vi "ResonanceScanner.vi"() -> ()   [LabVIEW 2012]
uses:
  <vilib>/Platform/TimedLoop/XDataNode/timing_clust.ctl
  <vilib>/Platform/TimedLoop/XDataNode/nitl_modes.ctl
  <vilib>/Platform/TimedLoop/XDataNode/wakeup.ctl
  <vilib>/rvi/eio/common/nirviEmuTemplateMethod_errors.vi
  <vilib>/rvi/FIFO/Fifo_Resource/nirvififoEmulationSetSize.vi
  <vilib>/rvi/DataTransferAndStorage/Container/Common/niFpgaContainerGetUniqueNameForEmu.vi
  <vilib>/rvi/Emulation/niFpgaSctlEmulationRegisterWithScheduler.vi
  <vilib>/rvi/errors/niFpgaSetErrorForExecOnDevCompSimple.vi
  <vilib>/rvi/eio/common/nirviEmuReportErrorAndStop.vi
  <vilib>/rvi/Emulation/niFpgaSctlEmulationFifoFullMgr.vi
  <vilib>/rvi/Emulation/niFpgaSctlEmulationResourceMgr.vi
  <vilib>/rvi/Emulation/niFpgaSctlEmulationScheduler.vi
  <vilib>/rvi/interface/RandomDataEmulation/nirviRandomDataFPGAFIFO.vi
  <vilib>/rvi/interface/RandomDataEmulation/niFpgaRandomDataHandleErrors.vi
  <vilib>/rvi/Emulation/niFpgaSctlEmulationGlobalWrite.vi
  <vilib>/Platform/TimedLoop/XDataNode/XDataNode.xnode
  <vilib>/eio/EIONode/EIONode.xnode
  <vilib>/rvi/DataTransferAndStorage/Container/XNode/niFpgaContainer.xnode
  <vilib>/rvi/FIFO/Fifo_Resource/nirvififoEmulationClear.vi
  <vilib>/rvi/FXPMathLib/basic elements/FxpDiscreteDelay/XNode/nifxpmath_DiscreteDelay.xnode
  <vilib>/rvi/FIFO/Fifo_Resource/nirvififoEmulationWrite.vi
  <vilib>/rvi/FIFO/Fifo_Resource/nirvififoEmulationRead.vi
  <vilib>/rvi/interface/RandomDataEmulation/nirviRandomDataFpgaReadWriteTemplate.vi
  <vilib>/Platform/TimedLoop/XDataNode/XDNodeRunTimeDep.lvlib
panel:
  in  "Scanner delay":i16=10000
  out "Pixel finished?":bool
  out "Resonance Trigger":bool
  in  "Baselinex8 Ch2":u16
  in  "Baselinex8 Ch1":u16
  in  "Clear Interloop FIFO":bool
  out "InterloopFIFO Timeout":bool
  out "ToHostCh2FIFO Overflow":bool
  out "ToHostCh1FIFO Overflow":bool
  out "Pixel counter":u32
  in  "Wait for trigger":bool
  in  "Acquire":bool
  in  "Acquire continuously":bool=TRUE
  in  "Requested pixels":u32=100000
  out "InterloopFIFO Overflow":bool
  out "Acquiring":bool
  out "IO Module\\AI Over Range":bool
  in  "Samples per pixel":u32=10000 caption="Samples per pixel Acq"
  in  "Samples per line":u32=10000 caption="Samples per pixel Acq"
  out "Configured?":bool
  # "5751 IO module configuration"
  # "Analog integrator"
  # "Acquisition control"
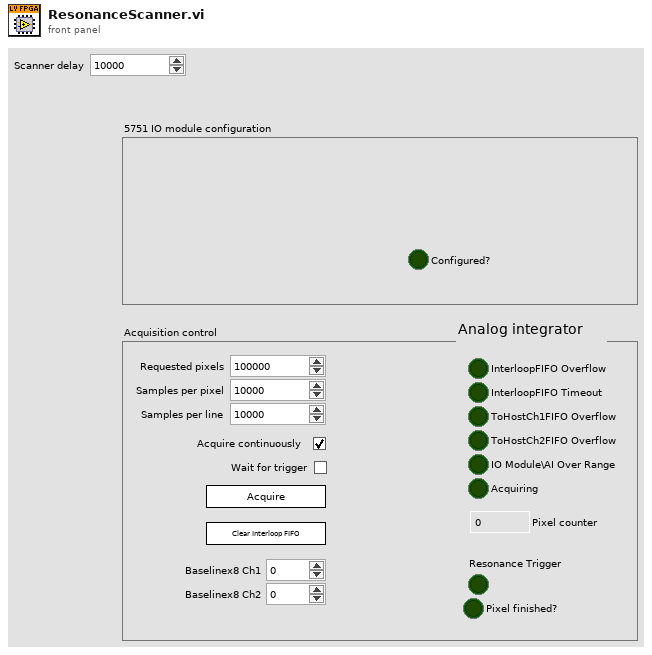
[diagram p1: front panel]
types:
  T1 = typedef "XDNodeRunTimeDep.lvlib/timing_clust.ctl" = cluster{"Expected End [f-1]":u64, "Actual End [f-1]":u64, "Finished Late? [f-1]":bool, "Expected End [i-1]":u64, "Actual End [i-1]":u64, "Finished Late? [i-1]":bool, "Expected Start [i]":u64, "Actual Start [i]":u64, "Expected Start [f]":u64, "Actual Start [f]":u64, "Source Name":string, "Structure Name":string, "Period":i64, "Deadline":i64, "Offset":i64, "Start":i64, "Priority":i32, "Timeout":i32, "Mode":T2, "Wakeup Reason":T3, "Error":errorcluster, "Source Type":string, "Secondary Source Type":string, "Global End Time":u64, "Global Start Time":u64, "Frame Duration":u64, "Iteration Duration":u64, "Assigned CPU":i32, "I/O Scan Engine Mode":u32}
  T2 = typedef "XDNodeRunTimeDep.lvlib/nitl_modes.ctl" = enum32{"No Change", "Process missed periods, maintain original phase", "Discard missed periods, maintain original phase", "Process missed periods, ignore original phase", "Discard missed periods, ignore original phase"}
  T3 = typedef "XDNodeRunTimeDep.lvlib/wakeup.ctl" = enum32{"Normal", "Aborted", "Asynchronous wakeup", "Timing source error", "Timed loop error", "Timeout"}
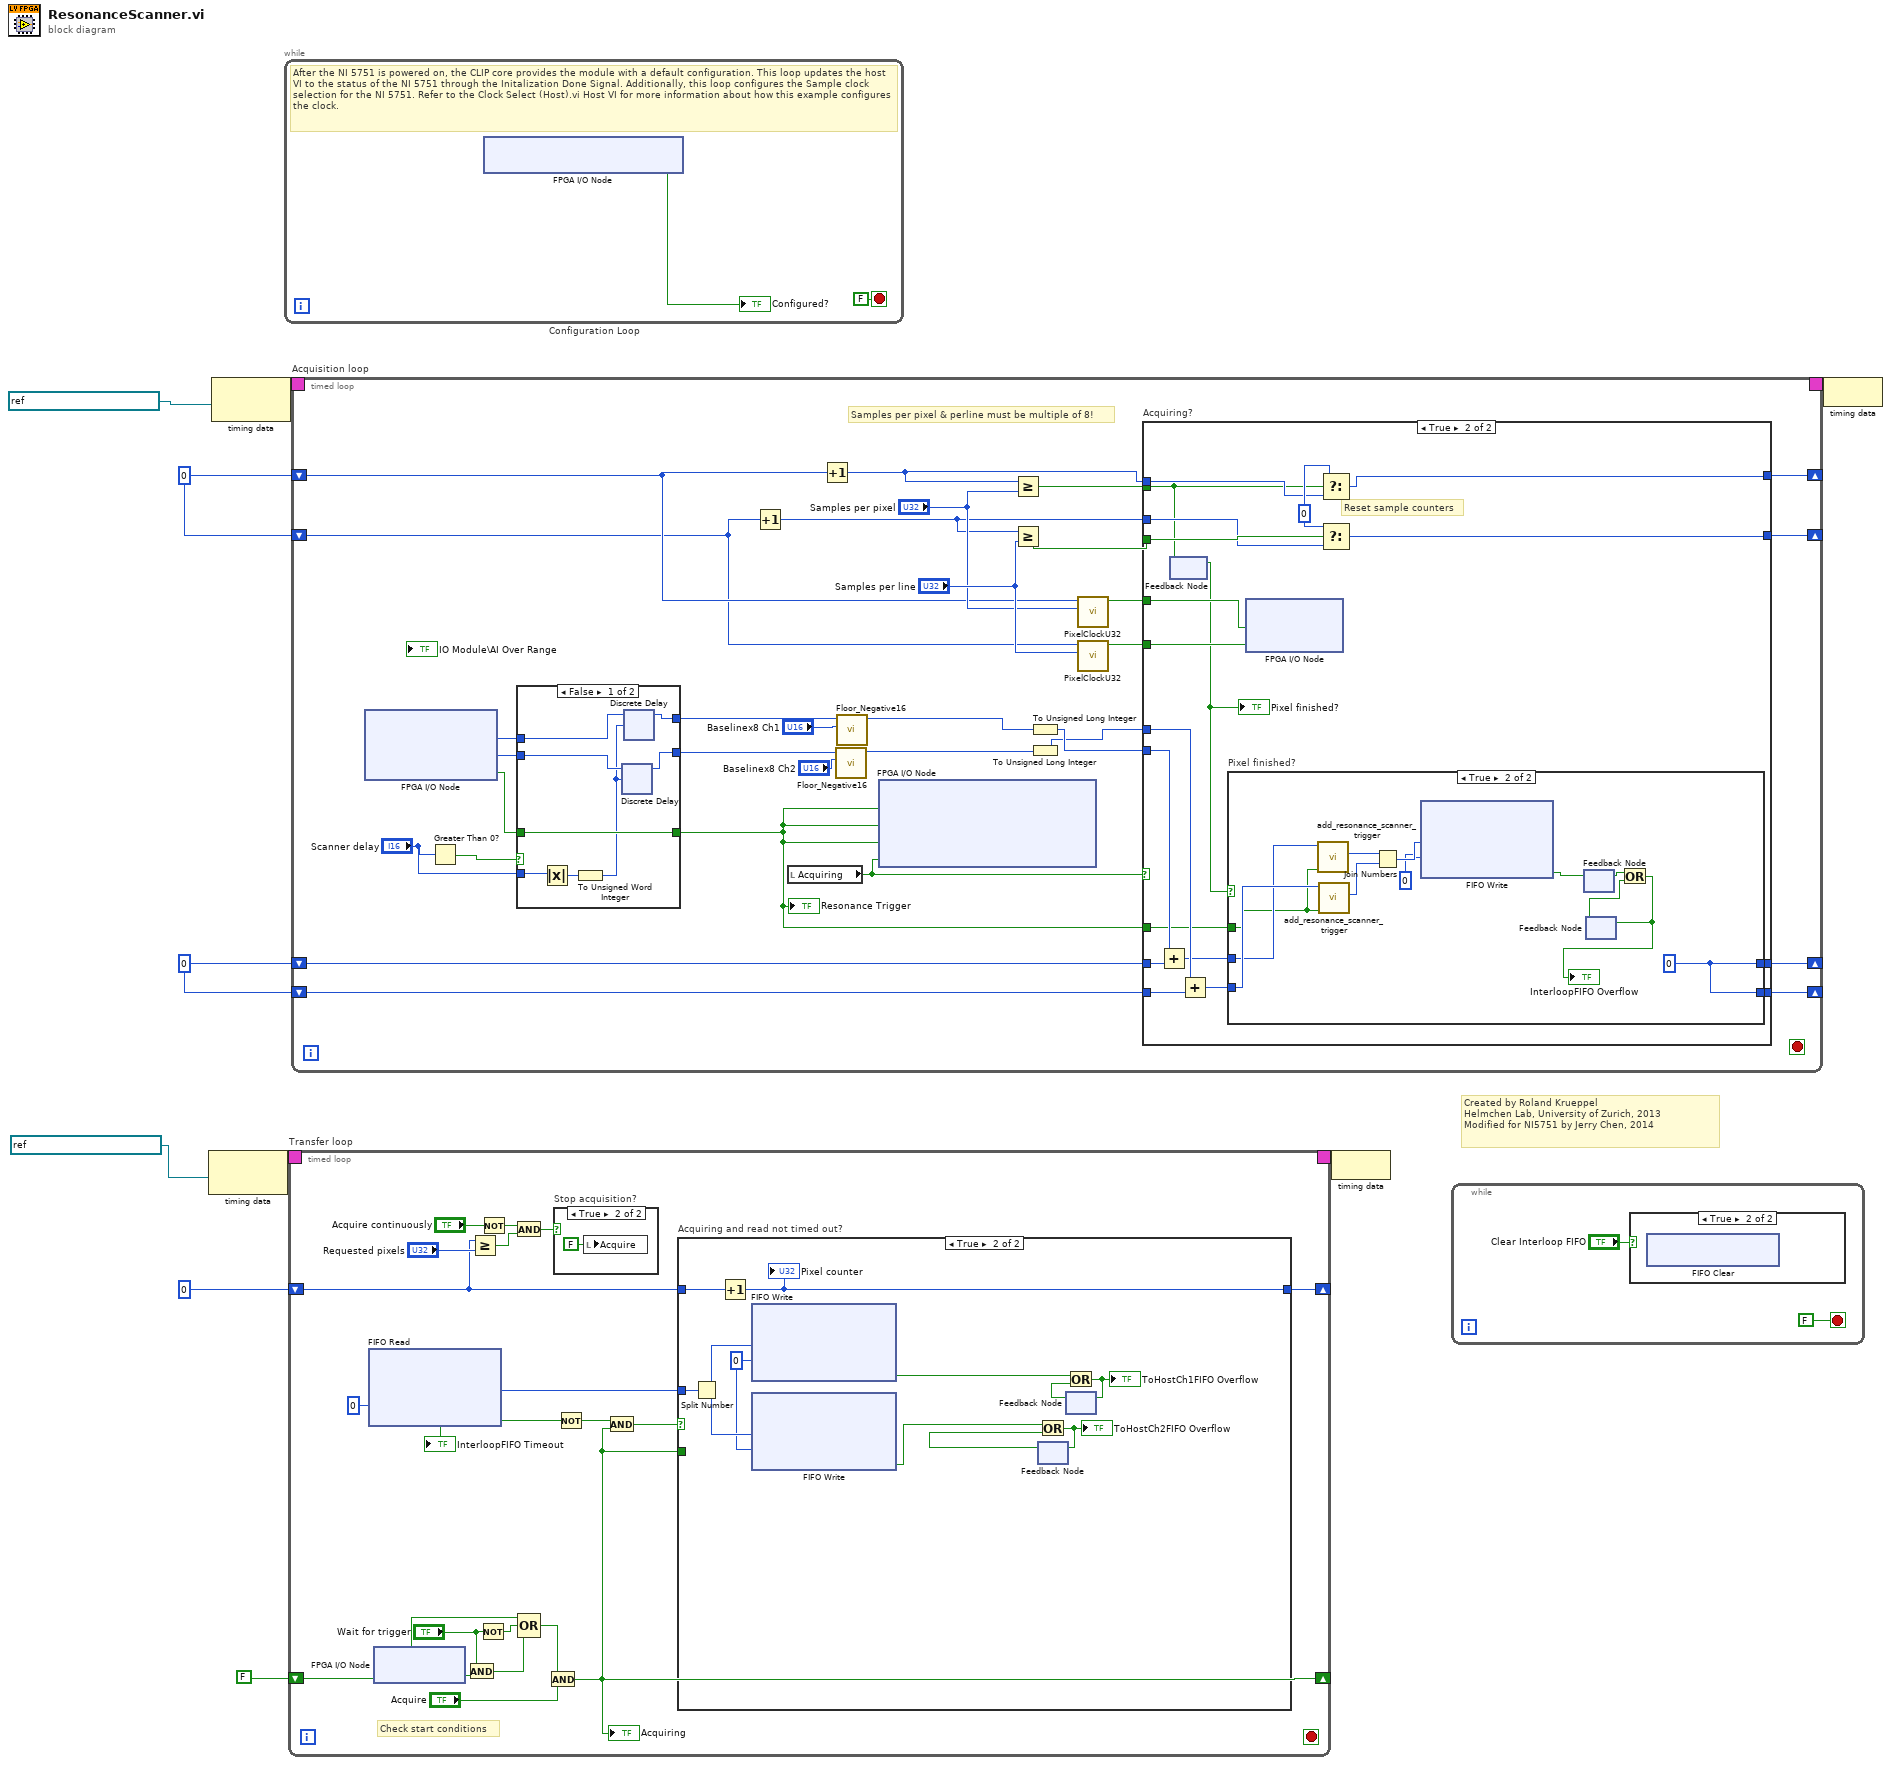
[diagram p0: block diagram]
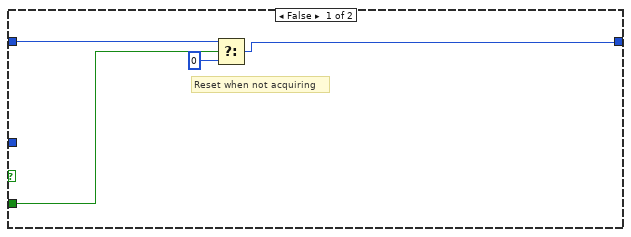
[diagram p4: hidden frame]
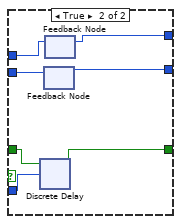
[diagram p5: hidden frame]
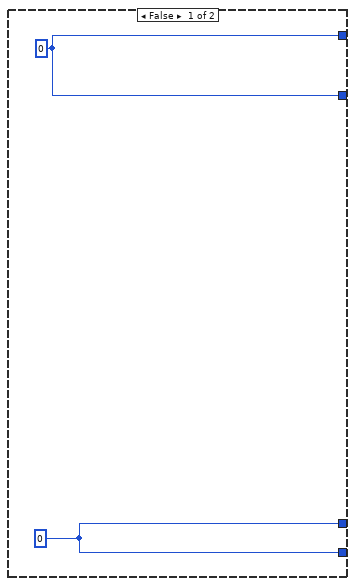
[diagram p6: hidden frame]
diagram:
  w7 = u32 0
  w8 = u32 0 ("t")
  # "Created by Roland Krueppel\nHelmchen Lab, University of Zurich, 2013\nModified for NI5751 by Jerry Chen, 2014"
  n1 = node-c288(refnum<k21> "40 MHz Onboard Clock" ("Source Name")) -> (w6:T1)
  n2 = node-c288(refnum<k21> "40 MHz Onboard Clock" ("Source Name")) -> (w10:T1)
  n3 = while "Configuration Loop" {
    stop <- FALSE stop-if-true
    # "After the NI 5751 is powered on, the CLIP core provides the module with a default configuration. This loop updates the host VI to the status of the NI 5751 through the Initalization Done Signal. Additionally, this loop configures the Sample clock selection for the NI 5751. Refer to the Clock Select (Host).vi Host VI for more information about how this example configures the clock."
    n4 = xnode "FPGA I/O Node"() -> ("IO Module\\Initialization Done"=→"Configured?":bool)  [unwired: 1 in, 1 out]
  }
  n5 = timed-loop "Transfer loop" {
    timing: w6 -> [_]
    timing-out: [_] -> w5
    shift-right: [w15] -> _
    shift-left: u32 0 -> [w16]
    shift-right: [w14] -> _
    shift-left: FALSE -> [w22]
    stop <- _ stop-if-true
    # "Check start conditions"
    n6 = xnode ("FIFO Read")("Timeout"=0) -> ("Element"=w17:u64, "Timed Out?"=w21:bool)  [unwired: 1 in, 1 out]
    "InterloopFIFO Timeout" <- w21
    n7 = xnode "FPGA I/O Node"() -> ("TriggerIn"=w27:bool)  [unwired: 1 in, 1 out]
    n8 = And(x="Wait for trigger", y=w27) -> (x .and. y?=w24:bool)
    n9 = Greater Or Equal?(x=w16, y="Requested pixels") -> (x >= y?=w29:bool)
    n10 = Not(x="Wait for trigger") -> (.not. x?=w25:bool)
    n11 = Not(x="Acquire continuously") -> (.not. x?=w30:bool)
    n12 = And(x=w30, y=w29) -> (x .and. y?=w19:bool)
    n13 = Compound Arithmetic op=OR(w22, w25, w24) -> (w23:bool)
    n14 = And(x=w23, y="Acquire") -> (x .and. y?=w14:bool)
    "Acquiring" <- w14
    n15 = case "Stop acquisition?" shown="True" w19 {
      frame False {
      }
      frame True {
        n16 = local write "Acquire"(FALSE ("Acquire")) -> ()
      }
    }
    n17 = Not(x=w21) -> (.not. x?=w20:bool)
    n18 = And(x=w20, y=w14) -> (x .and. y?=w18:bool)
    n19 = case "Acquiring and read not timed out?" shown="True" w18 {
      tunnel: w17 -> [_ w49]
      tunnel: w16 -> [w36 w45]
      tunnel: [w35 w44] -> w15
      tunnel: w14 -> [w37 _]
      frame False {
        # "Reset when not acquiring"
        n20 = Select(t=w36, s=w37, f=u32 0) -> (s? t:f=w35:u32)
      }
      frame True {
        w46 = 0 ("Timeout")
        n21 = Split Number(x=w49) -> (hi(x)=w48:u32, lo(x)=w47:u32)
        n22 = Increment(x=w45) -> (x+1=w44:u32)
        "Pixel counter" <- w44
        n23 = xnode ("FIFO Write")("Element"=w48, "Timeout"=w46) -> ("Timed Out?"=w42:bool)  [unwired: 1 in, 1 out]
        n24 = xnode ("FIFO Write")("Element"=w47, "Timeout"=w46) -> ("Timed Out?"=w39:bool)  [unwired: 1 in, 1 out]
        n25 = feedback #1() -> (w38:bool)  [unwired: 1 in]
        n26 = Or(x=w39, y=w38) -> (x .or. y?=w40:bool)
        "ToHostCh2FIFO Overflow" <- w40
        n27 = feedback-in #1(w40) -> ()
        n28 = feedback #2() -> (w41:bool)  [unwired: 1 in]
        n29 = Or(x=w42, y=w41) -> (x .or. y?=w43:bool)
        "ToHostCh1FIFO Overflow" <- w43
        n30 = feedback-in #2(w43) -> ()
      }
    }
  }
  n31 = timed-loop "Acquisition loop" {
    timing: w10 -> [_]
    timing-out: [_] -> w9
    shift-right: [w81] -> _
    shift-left: w8 -> [w62]
    shift-right: [w82] -> _
    shift-left: w8 -> [w64]
    shift-right: [w78] -> _
    shift-left: w7 -> [w80]
    shift-right: [w77] -> _
    shift-left: w7 -> [w79]
    stop <- _ stop-if-true
    # "Samples per pixel & perline must be multiple of 8!"
    n32 = xnode "FPGA I/O Node"() -> ("IO Module\\AI A0"=w56:i16, "IO Module\\AI A2"=w55:i16, "IO Module\\DI 0"=w60:bool)  [unwired: 3 in, 3 out]
    n33 = Greater Than 0?(x="Scanner delay") -> (x > 0?=w52:bool)
    n34 = case shown="False" w52 {
      tunnel: w60 -> [w86 w97]
      tunnel: [w86 w96] -> w58
      tunnel: "Scanner delay" -> [w85 w95]
      tunnel: w56 -> [w89 w94]
      tunnel: w55 -> [w90 w93]
      tunnel: [w87 w92] -> w54
      tunnel: [w88 w91] -> w53
      frame False {
        n35 = Absolute Value(x=w85) -> (abs(x)=w84:i16)
        n36 = To Unsigned Word Integer(number=w84) -> (unsigned 16bit integer=w83:u16)
        n37 = xnode "Discrete Delay"("D"=w90, "n-1[0..511]"=w83) -> ("Q"=w87:i16)
        n38 = xnode "Discrete Delay"("D"=w89, "n-1[0..511]"=w83) -> ("Q"=w88:i16)
      }
      frame True {
        n39 = xnode ("Discrete Delay")("D"=w97, "n-1[0..511]"=w95) -> ("Q"=w96:bool)
        n40 = feedback #3() -> (w92:i16)  [unwired: 1 in]
        n41 = feedback-in #3(w93) -> ()
        n42 = feedback #4() -> (w91:i16)  [unwired: 1 in]
        n43 = feedback-in #4(w94) -> ()
      }
    }
    "Resonance Trigger" <- w58
    n44 = Increment(x=w62) -> (x+1=w61:u32)
    n45 = local read "Acquiring"() -> (w59:bool)
    n46 = Increment(x=w64) -> (x+1=w63:u32)
    n47 = call "Floor_Negative16.vi"("Baseline U16"="Baselinex8 Ch2", "Input Value"=w54) -> ("Output Value"=w69:u16)  [unwired: 9 in]
    n48 = call "Floor_Negative16.vi"("Baseline U16"="Baselinex8 Ch1", "Input Value"=w53) -> ("Output Value"=w70:u16)  [unwired: 9 in]
    n49 = xnode "FPGA I/O Node"("IO Module\\D0 2"=w58, "IO Module\\D0 3"=w58, "IO Module\\D0 4"=w58, "IO Module\\Digital Output Enable"=w59) -> ()  [unwired: 4 in, 4 out]
    n50 = Greater Or Equal?(x=w63, y="Samples per pixel") -> (x >= y?=w72:bool)
    n51 = Greater Or Equal?(x=w61, y="Samples per line") -> (x >= y?=w71:bool)
    n52 = To Unsigned Long Integer(number=w70) -> (unsigned 32bit integer=w66:u32)
    n53 = To Unsigned Long Integer(number=w69) -> (unsigned 32bit integer=w65:u32)
    n54 = call "PixelClockU32.vi"("Samples per pixel"="Samples per pixel", "Sample counter"=w64) -> ("Pixel clock"=w74:bool)  [unwired: 9 in]
    n55 = call "PixelClockU32.vi"("Samples per pixel"="Samples per line", "Sample counter"=w62) -> ("Pixel clock"=w73:bool)  [unwired: 9 in]
    n56 = case "Acquiring?" shown="True" w59 {
      tunnel: [w99 w117] -> w82
      tunnel: [w99 w116] -> w81
      tunnel: w66 -> [_ w114]
      tunnel: w80 -> [_ w115]
      tunnel: w79 -> [_ w113]
      tunnel: w65 -> [_ w112]
      tunnel: [w98 w109] -> w78
      tunnel: [w98 w108] -> w77
      tunnel: w72 -> [_ w102]
      tunnel: w71 -> [_ w107]
      tunnel: w63 -> [_ w106]
      tunnel: w61 -> [_ w105]
      tunnel: w74 -> [_ w104]
      tunnel: w73 -> [_ w103]
      tunnel: w58 -> [_ w101]
      frame False {
        w98 = u32 0
        w99 = u16 0 ("t")
      }
      frame True {
        w118 = u32 0 ("t")
        # "Reset sample counters"
        n57 = Add(x=w114, y=w115) -> (x+y=w110:u32)
        n58 = feedback #5() -> (w100:bool)  [unwired: 1 in]
        "Pixel finished?" <- w100
        n59 = feedback-in #5(w102) -> ()
        n60 = Add(x=w112, y=w113) -> (x+y=w111:u32)
        n61 = case "Pixel finished?" shown="True" w100 {
          tunnel: w111 -> [w119 w125]
          tunnel: w110 -> [w120 w124]
          tunnel: [w120 w128] -> w109
          tunnel: [w119 w128] -> w108
          tunnel: w101 -> [_ w123]
          frame False {
          }
          frame True {
            w128 = u32 0
            n62 = call "add_resonance_scanner_trigger.vi"("Trigger"=w123, "Input"=w124) -> ("Output"=w122:u32)  [unwired: 9 in]
            n63 = call "add_resonance_scanner_trigger.vi"("Trigger"=w123, "Input"=w125) -> ("Output"=w121:u32)  [unwired: 9 in]
            n64 = Join Numbers(hi=w122, lo=w121) -> ((hi.lo)=w132:u64)
            n65 = xnode ("FIFO Write")("Element"=w132, "Timeout"=0) -> ("Timed Out?"=w126:bool)  [unwired: 1 in, 1 out]
            n66 = feedback-in #6(w126) -> ()
            n67 = feedback #6() -> (w127:bool)  [unwired: 1 in]
            n68 = feedback #7() -> (w129:bool)  [unwired: 1 in]
            n69 = Or(x=w127, y=w129) -> (x .or. y?=w130:bool)
            "InterloopFIFO Overflow" <- w130
            n70 = feedback-in #7(w130) -> ()
          }
        }
        n71 = xnode "FPGA I/O Node"("PixelClock"=w104, "LineClock"=w103) -> ()  [unwired: 2 in, 2 out]
        n72 = Select(t=w118, s=w102, f=w106) -> (s? t:f=w117:u32)
        n73 = Select(t=w118, s=w107, f=w105) -> (s? t:f=w116:u32)
      }
    }
  }
  n74 = node-c288(w5) -> ()
  n75 = while {
    stop <- FALSE stop-if-true
    n76 = case shown="True" "Clear Interloop FIFO" {
      frame False {
      }
      frame True {
        n77 = xnode ("FIFO Clear")() -> ()  [unwired: 1 in, 1 out]
      }
    }
  }
  n78 = node-c288(w9) -> ()
